vi "全局.vi"() -> ()   [LabVIEW 2018]
panel:
  in  "拉压力调零":dbl
  in  "球阀预调确认":dbl
  in  "球阀开口度 预调":dbl
  in  "球阀反馈值":dbl
  in  "自动模式":dbl
  out "布尔 2":bool
  in  "cns":dbl
  in  "放气":dbl
  in  "试验结束":dbl
  in  "放气延迟":dbl
  in  "保压时间固定":dbl
  in  "不保压":dbl
  in  "紧急停止":dbl
  in  "测":dbl
  out "X体横向位移2":dbl
  out "X体横向位移1":dbl
  out "周向转动摩擦力2":dbl
  out "周向转动摩擦力1":dbl
  out "横向拉压力2":dbl
  out "横向拉压力1":dbl
  out "容器压力2":dbl
  out "容器压力1":dbl
  out "管道压力2":dbl
  out "管道压力1":dbl
  in  "保压时间":dbl
  in  "电磁阀2":dbl
  in  "电磁阀1":dbl
  in  "手动模式":dbl
  in  "结束保存":dbl
  in  "数据保存":dbl
  in  "采样时间":dbl
  out "布尔":bool
  in  "球阀 开口度":dbl
  in  "D":dbl
  in  "I":dbl
  in  "P":dbl
  in  "容器放气":dbl
  in  "保压模式":dbl
  in  "实验所需气压":dbl
  in  "全部放气":dbl
  in  "采样频率":dbl
  in  "程序运行":dbl
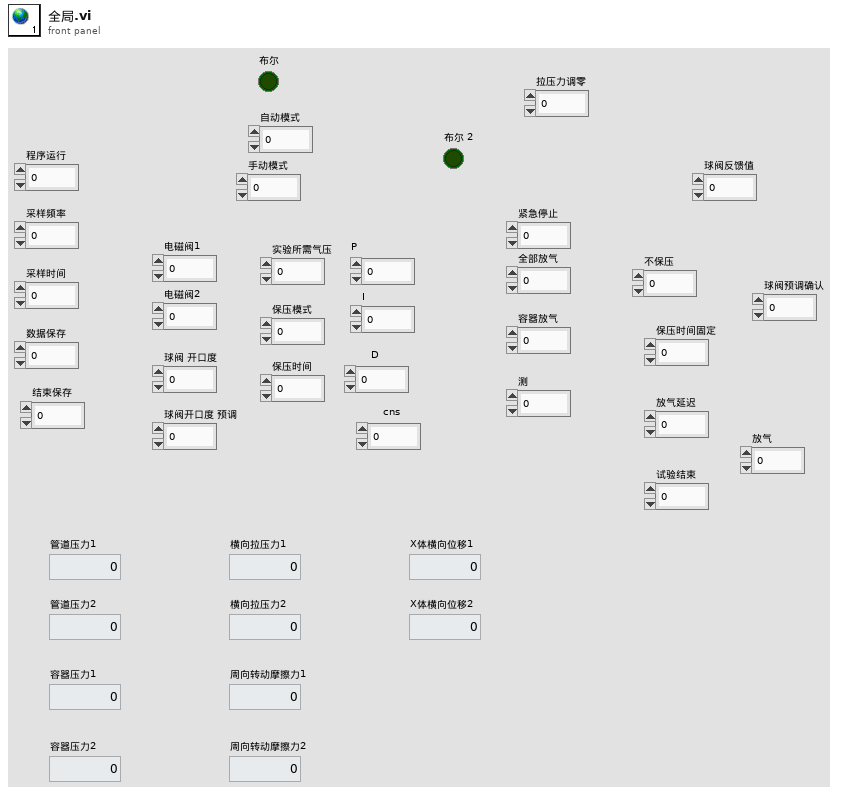
[diagram p1: front panel]
diagram:
